vi "getDeviceArray.vi"(8 "error in (no error)":errorcluster, 11 "ScriptListCompiler.lvclass in":refnum<class "ScriptListCompiler.lvclass">) -> (0 "error out":errorcluster, 2 "DeviceArray":refnum<class "DeviceArray.lvclass">, 3 "ScriptListCompiler.lvclass out":refnum<class "ScriptListCompiler.lvclass">)   [LabVIEW 2011, in "Compiler.lvlib" / "ScriptListCompiler.lvclass"]
uses:
  ScriptListCompiler.lvclass
  DatabaseHelpers/Database Objects/DeviceArray/DeviceArray.lvclass
  ScriptListCompiler.lvclass/ScriptListCompiler.ctl
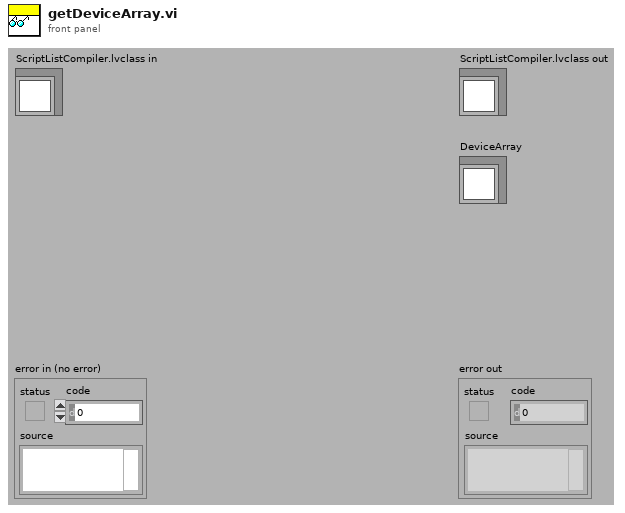
[diagram p1: front panel]
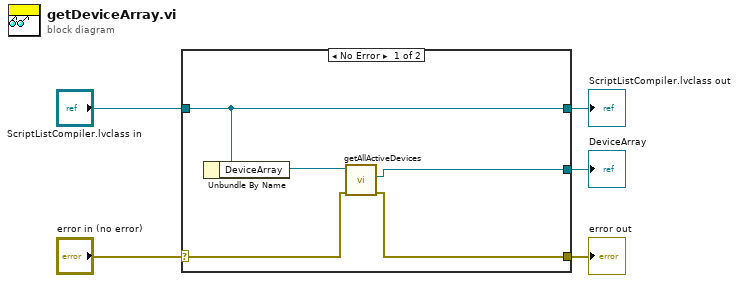
[diagram p0: block diagram]
diagram:
  n1 = case shown="No Error" "error in (no error)" {
    selector: "error in (no error)" -> [w7 w11]
    tunnel: [w6 w11] -> w4
    tunnel: [w10 w12] -> w2
    tunnel: "ScriptListCompiler.lvclass in" -> [w10 w12]
    tunnel: [w8 _] -> w1
    frame No Error {
      n2 = Unbundle By Name(w10) -> ("DeviceArray"=w9:refnum<class "DeviceArray.lvclass">)
      n3 = call "getAllActiveDevices.vi"("error in (no error)"=w7, "DeviceArray in"=w9) -> ("error out"=w6:errorcluster, "DeviceArray"=w8:refnum<class "DeviceArray.lvclass">)  [unwired: 7 in, 1 out]
    }
    frame Error {
    }
  }
  "error out" <- w4
  "ScriptListCompiler.lvclass out" <- w2
  "DeviceArray" <- w1
